vi "ReadOrDestroyStream.vi"(7 "EndpointName":string, 8 "error in (no error)":errorcluster, 9 "Connected":bool, 10 "IP Address":string, 11 "Refnum in":refnum<k21>) -> (0 "error out":errorcluster, 2 "data out":T1[](array[typedef]), 3 "Refnum":refnum<k21>)   [LabVIEW 2018]
uses:
  Win_Controls/Enums/Win_Rcv_Enum.ctl
  Win_Controls/Clust/Win_Read_Clust.ctl
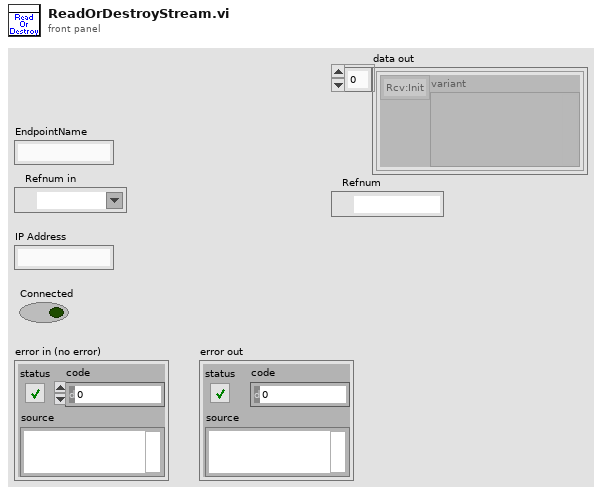
[diagram p1: front panel]
types:
  T1 = typedef "Win_Read_Clust.ctl" = cluster{T2, "variant":variant}
  T2 = typedef "Win_Rcv_Enum.ctl" = enum16{"Rcv:Init", "Rcv:Read", "Rcv:Log", "Rcv:FromMast", "Rcv:FromSlav"}
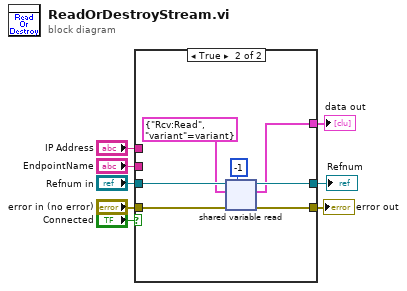
[diagram p0: block diagram]
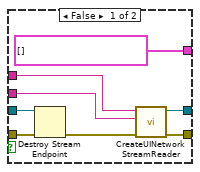
[diagram p2: hidden frame]
diagram:
  n1 = case shown="True" "Connected" {
    tunnel: [w15 w20] -> w1
    tunnel: [w16 w21] -> w4
    tunnel: "Refnum in" -> [w12 w23]
    tunnel: "error in (no error)" -> [w14 w22]
    tunnel: "IP Address" -> [w11 _]
    tunnel: "EndpointName" -> [w10 _]
    tunnel: [T1[] [] w17] -> w2
    frame False {
      n2 = Destroy Stream Endpoint(8:w14, 11:w12) -> (0:w13:errorcluster)
      n3 = call "CreateUINetworkStreamReader.vi"("ErrorIn"=w13, "ReaderName"=w10, "IPAddress"=w11) -> ("ErrorOut"=w16:errorcluster, "reader endpoint"=w15:refnum<k21>)  [unwired: 7 in]
    }
    frame True {
      n4 = shared-variable-read(w23, w22, -1 ("# elements"), T1 {enum."Rcv:Read", "variant"=variant}) -> (w20:refnum<k21>, w21:errorcluster, w17:T1[])  [unwired: 1 in, 1 out]
    }
  }
  "error out" <- w4
  "data out" <- w2
  "Refnum" <- w1
